vi "DeltaRT_us.vi"(7 "Initial delta time":i32 caption="Initial delta time (0) [µs]", 11 "Error in":errorcluster caption="Error in (no error)") -> (8 "Time since last call":i32 caption="Time since last call [µs]", 15 "Error out":errorcluster)   [LabVIEW 2017, in "GPTiming.lvlib"]
doc: "Calculates the elapsed <B>Time since last call</B> of the particular instance of this VI. This can be used in a loop for instance to calculate the time-step since last cycle.\n\nThe very first time this VI is called there has passed zero time since last call (as there was no last call), so by default it will return 0 in <B>Time since last call</B> in this case. Optionally you can wire another value to <B>Initial delta time</B> to make this VI return that value instead on the first call. <B>Initial delta time</B> will not affect consecutive calls in any way, only the very first call.\n\nThis VI uses the Real-Time microsecond tick counter and will be able to count time-steps of up to 2^31-1 microseconds (almost 36 minutes).\n\nThis VI is inlined. <B>Error in</B> is wired straight through to <B>Error out</B> to enable optional dataflow dependency (offering control of when the time-step is calculated at).\n\nSteen Schmidt\nGPower\n8/12 2013"
uses:
  GPTiming.lvlib
panel:
  # "Copyright © 2013\nGPower\nSee enclosed license file for terms and conditions"
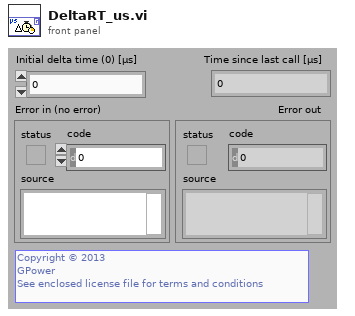
[diagram p1: front panel]
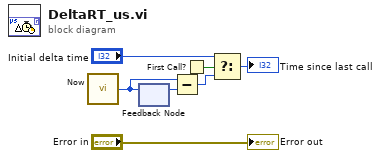
[diagram p0: block diagram]
diagram:
  n1 = call "Now"() -> ("Tick Count(uSec)"=w2:u32)
  n2 = feedback-in #1(w2) -> ()
  n3 = feedback #1() -> (w7:u32)  [unwired: 1 in]
  n4 = Subtract(x=w2, y=w7) -> (x-y=w4:u32)
  n5 = First Call?() -> (First Call?: T/F=w6:bool)
  n6 = Select(t="Initial delta time", s=w6, f=w4) -> (s? t:f=→"Time since last call":u32)
  "Error out" <- "Error in"
